vi "Read Probe Attenuation.vi"(8 "error in (no error)":errorcluster, 10 "Channel (0: Channel 1)":u16(ring) items=["Channel 1", "Channel 2", "Channel 3", "Channel 4"], 11 "VISA resource name":refnum<visa-resource-name>) -> (0 "error out":errorcluster, 2 "Attenuation":dbl, 3 "VISA resource name out":refnum<visa-resource-name>)   [LabVIEW 2015, in "LeCroy Wave Series.lvlib"]
doc: "Read the attenuation factor of the specified channel."
uses:
  <instrlib>/LeCroy Wave Series/LeCroy Wave Series.lvlib
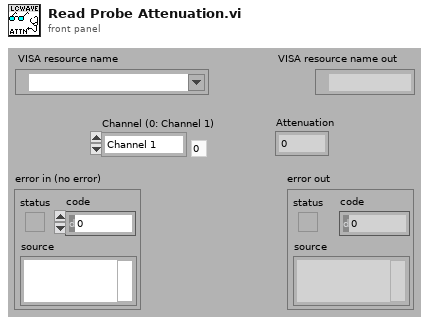
[diagram p1: front panel]
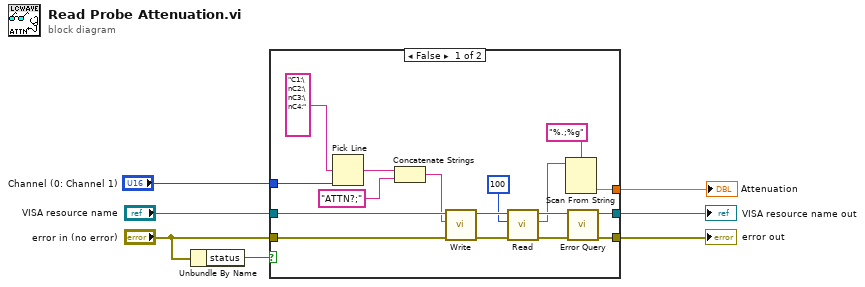
[diagram p0: block diagram]
diagram:
  n1 = Unbundle By Name("error in (no error)") -> ("status"=w1:bool)
  n2 = case shown="False" w1 {
    tunnel: "VISA resource name" -> [w21 w26]
    tunnel: "error in (no error)" -> [w20 w25]
    tunnel: [w17 w26] -> w6
    tunnel: [w16 w25] -> w5
    tunnel: "Channel (0: Channel 1)" -> [w14 _]
    tunnel: [w8 _] -> w3
    frame False {
      n3 = Pick Line(multi-line string="C1:\nC2:\nC3:\nC4:", line index=w14) -> (output string=w13:string)  [unwired: 1 in]
      n4 = Concatenate Strings(w13, "ATTN?;") -> (w11:string)
      n5 = call <instrlib>:"Write.vi"("error in (no error)"=w20, "Write Buffer"=w11, "VISA resource name"=w21) -> ("error out"=w24:errorcluster, "VISA resource name out"=w23:refnum<visa-resource-name>)  [unwired: 6 in, 1 out]
      n6 = call <instrlib>:"Read.vi"("error in (no error)"=w24, "Byte Count"=u32 100, "VISA resource name"=w23) -> ("error out"=w18:errorcluster, "Read Buffer"=w9:string, "VISA resource name out"=w19:refnum<visa-resource-name>)  [unwired: 5 in, 1 out]
      n7 = Scan From String(format string="%.;%g", input string=w9) -> (output 1=w8:dbl)  [unwired: 3 in, 3 out]
      n8 = call <instrlib>:"Error Query.vi"("error in (no error)"=w18, "VISA resource name"=w19) -> ("error out"=w16:errorcluster, "VISA resource name out"=w17:refnum<visa-resource-name>)  [unwired: 6 in, 2 out]
    }
    frame True {
    }
  }
  "error out" <- w5
  "VISA resource name out" <- w6
  "Attenuation" <- w3
